vi "Test XYZ Table Stage Module All Axis.vi"() -> ()   [LabVIEW 2018]
uses:
  Hardware Mfg/Thorlabs Translation Stages/Controls/Translation Stage Cluster.ctl
  General/Controls/Translation Stage Types.ctl
  General/Controls/Translation Stage Parameters.ctl
  General/Controls/Set Get Controls.ctl
  Hardware Mfg/Thorlabs Translation Stages/Controls/Motion Translation Module Control.ctl
panel:
  in  "Table Stages":T1={"X Stage"={"Position"=0.0, "Is.Enabled?"=FALSE, "Is.Connected?"=FALSE, "Device SN"="45876425", "AccelerationMaximum"=0.0, "VelocityMaximum"=0.0, "Acceleration"=0.0, "Velocity"=0.0, "waitTimeout (ms)"=0, "Model"=enum."None", "Is.Homed?"=FALSE}, "Y Stage"={"Position"=0.0, "Is.Enabled?"=FALSE, "Is.Connected?"=FALSE, "Device SN"="45995820", "AccelerationMaximum"=0.0, "VelocityMaximum"=0.0, "Acceleration"=0.0, "Velocity"=0.0, "waitTimeout (ms)"=0, "Model"=enum."None", "Is.Homed?"=FALSE}, "Z Stage"={"Position"=0.0, "Is.Enabled?"=FALSE, "Is.Connected?"=FALSE, "Device SN"="49103464", "AccelerationMaximum"=0.0, "VelocityMaximum"=0.0, "Acceleration"=0.0, "Velocity"=0.0, "waitTimeout (ms)"=0, "Model"=enum."None", "Is.Homed?"=FALSE}}
  out "Cluster":T4
  in  "Z Pos":dbl caption="Position"
  in  "Y Pos":dbl caption="Position"
  in  "X Pos":dbl caption="Position"
  out "Error Out":errorcluster
  in  "Uninit":bool
  in  "Init":bool
  in  "Cancel Button":bool
  in  "Position":bool
  in  "Stop":bool
  in  "Home":bool
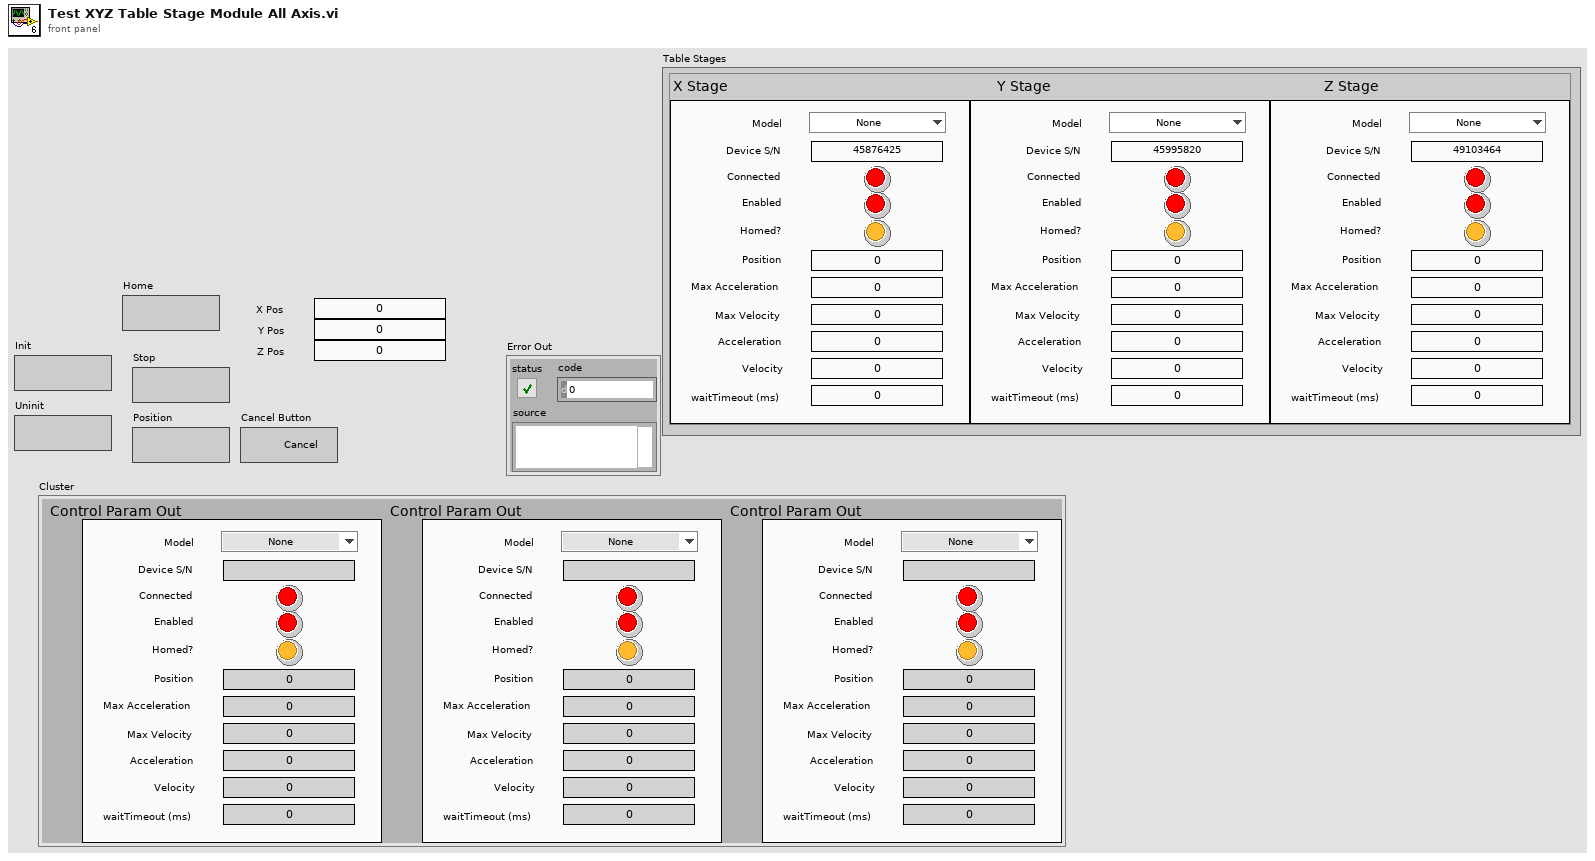
[diagram p1: front panel]
types:
  T1 = typedef "Translation Stage Parameters.ctl" = cluster{"X Stage":T2, "Y Stage":T2, "Z Stage":T2}
  T2 = typedef "Translation Stage Cluster.ctl" = cluster{"Position":dbl, "Is.Enabled?":bool, "Is.Connected?":bool, "Device SN":string, "AccelerationMaximum":dbl, "VelocityMaximum":dbl, "Acceleration":dbl, "Velocity":dbl, "waitTimeout (ms)":i32, "Model":T3, "Is.Homed?":bool}
  T3 = typedef "Translation Stage Types.ctl" = enum16{"None", "Thorlabs LTS", "Thorlabs MLJ"}
  T4 = cluster{"Control Param Out":T2, "Control Param Out":T2, "Control Param Out":T2}
  T5 = typedef "Motion Translation Module Control.ctl" = enum16{"Init", "Home", "Status", "Velocity/Accel", "Position", "Jog", "Stop", "Uninit", "Enable", "Disable"}
  T6 = typedef "Set Get Controls.ctl" = enum16{"Set", "Get"}
  T7 = typedef "System Parameters.ctl" = cluster{"Optical Parameters":T8, "Vibratome":T9, "Table Stages":T1, "Imaging Parameter":T10, "Galvo HW Parameters":cluster{"Analog Out Channel":tag, "Min Voltage":dbl, "Max Voltage":dbl, "Pixel Clock Source":tag, "Sample Rate":dbl, "Line Clock Out Ch":tag}, "Alazar parameters":T12, "Mosaic Paramter":cluster{"X Axis":cluster{"Start [mm]":dbl, "Steps [pts]":u16, "End [mm]":dbl}, "Y Axis":cluster{"Start [mm]":dbl, "Steps [pts]":u16, "End [mm]":dbl}, "Scan Pattern":enum16{"Uni-directional", "Bi-Directional", "Spiral Out", "Spiral In"}, "Overlap Options":cluster{"Overlap Type":enum16{"No Overlap", "X Only", "Y Only", "X and Y"}, "Percent Overlap":u8, "Justify":enum16{"Start", "Center", "End"}}}, "Vibratome Axis":cluster{"Start [mm]":dbl, "thick[mm]":dbl, "End [mm]":dbl}}
  T8 = typedef "Optical Parameters.ctl" = cluster{"Obj. Focal Length [mm]":dbl, "Scan Lens EFL[mm]":dbl, "Tube Lens EFL[mm]":dbl, "Galvo V Range (+/-)":dbl, "Galvo Max Half Angle [Deg]":dbl, "Max Galvo Range[%]":dbl}
  T9 = typedef "Vibratome Parameters.ctl" = cluster{"Z Bottom [mm]":dbl, "Pre Cut Dwell [s]":dbl, "Blade Frequency [RPM]":u16, "Slice Speed [mm/s]":dbl, "Post Cut Dwell [s]":dbl, "Ramp Time [s]":dbl, "Start X [mm]":dbl, "Start Y [mm]":dbl, "Slice Length [mm]":dbl, "Slice Axis":enum16{"X Axis", "Y Axis", "Z Axis"}, "Controller VISA Ref":refnum<visa-resource-name>}
  T10 = typedef "Imaging Parameters.ctl" = cluster{"Raster Scan Direction":T11, "Pixel Dwell Time [Clock Cycles]":u16, "Flyback Time [Clock Cycles]":u16, "XY Center [um]":cluster{"X":dbl, "Y":dbl}, "Pixel Step Size [um]":dbl, "XY Image Size":enum16{"32 x 32", "64 x 64", "128 x 128", "256 x 256", "512 x 512", "1024 x 1024", "2048 x 2048"}, "Custom":bool, "Custom Size":cluster{"X":u16, "Y":u16}, "Line Averages":u8}
  T11 = typedef "Scan Direction.ctl" = enum16{"Uni Directional", "Bi Directional", "None"}
  T12 = typedef "Alazar parameters.ctl" = cluster{"Trigger Settings":cluster{"General Trigger Settings":T13, "Trigger Engine 1":T14, "Trigger Engine 2":T14}, "Capture Clock":T15, "Device ID":T16, "Ch A Input Control":T17, "Ch B Input Control":T17, "Acq Settings":T18}
  T13 = typedef "General Trigger Settings.ctl" = cluster{"Trigger Operation":u32, "Coupling ID":u32, "Range ID":u32, "Delay":u32, "Timeout Ticks":u32, "Mode":u32, "Parameter":u32}
  T14 = typedef "Trigger Engine Controls.ctl" = cluster{"Trigger Engine":u32, "Source":u32, "Slope":u32, "Level":u32}
  T15 = typedef "Clock Controls.ctl" = cluster{"Sample Rate":u32, "Decimation":u32, "Source":u32, "Edge":u32}
  T16 = typedef "Alazar Device ID.ctl" = cluster{"System ID":u32, "Board ID":u32}
  T17 = typedef "Channel Input Controls.ctl" = cluster{"Channel":u8, "Coupling":u32, "Range":u32, "Impedance":u32}
  T18 = typedef "Alazar Acquisition Settings.ctl" = cluster{"Window Type":u32, "Record Length":u32, "Footer":u32, "Offset":u32, "Records Per Buffer":u32, "Samples per record":u32, "Records Count (Records/Acq)":u32, "Output Format":u32}
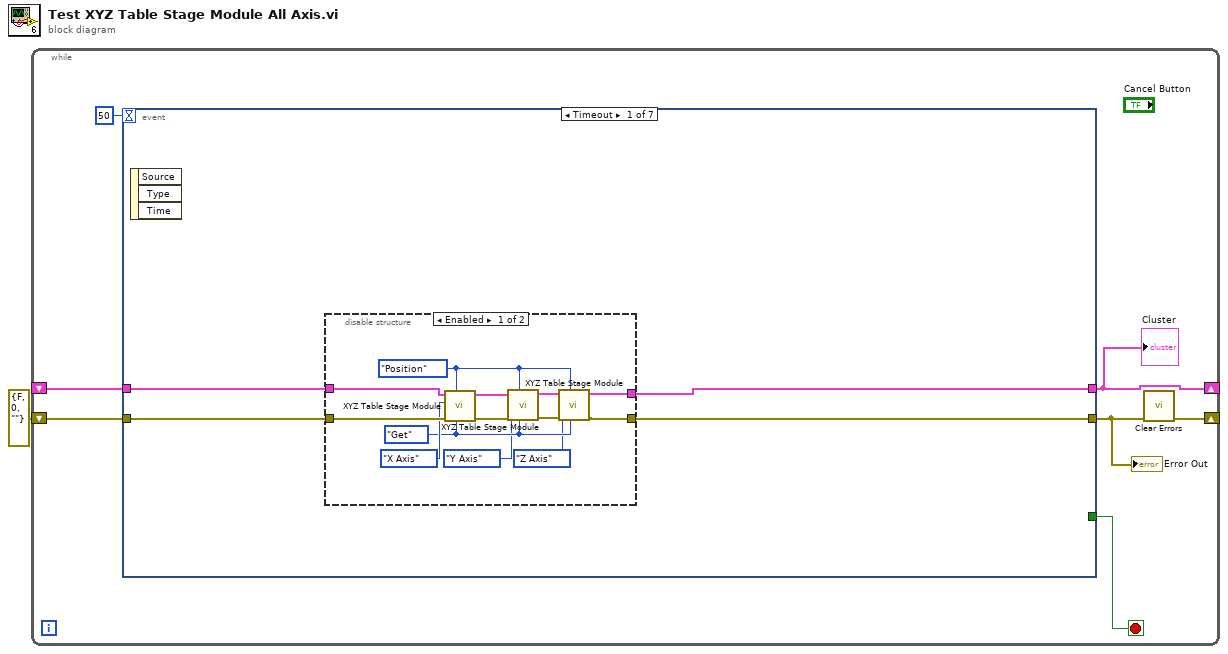
[diagram p0: block diagram]
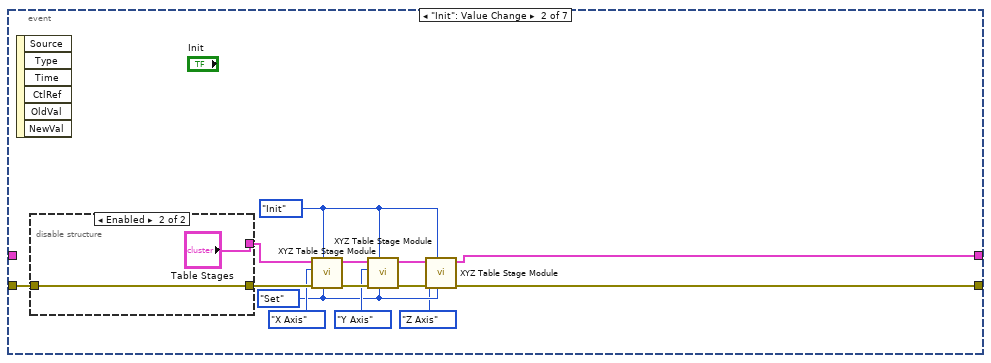
[diagram p3: hidden frame]
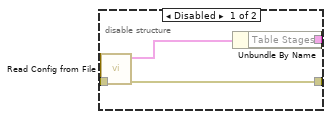
[diagram p4: hidden frame]
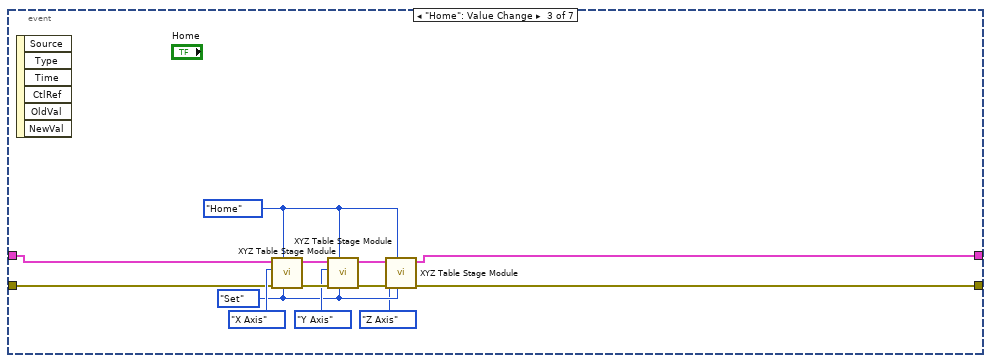
[diagram p5: hidden frame]
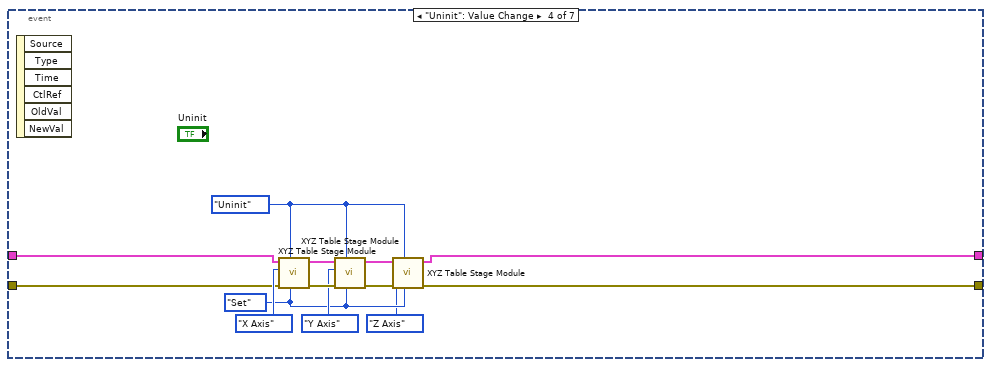
[diagram p6: hidden frame]
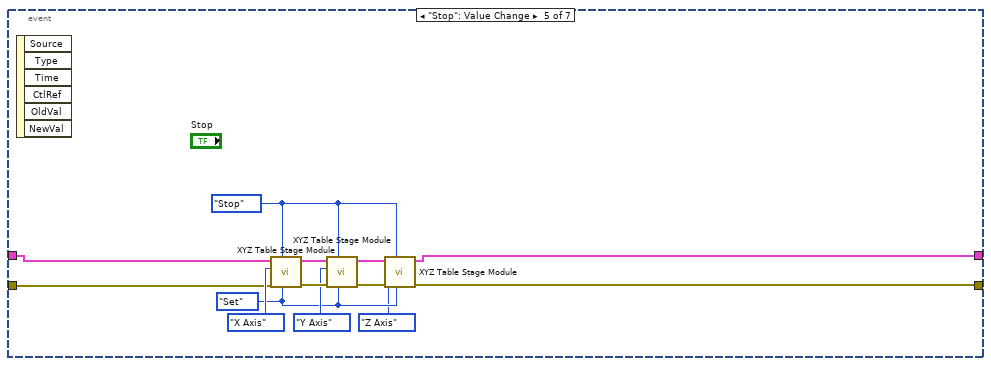
[diagram p7: hidden frame]
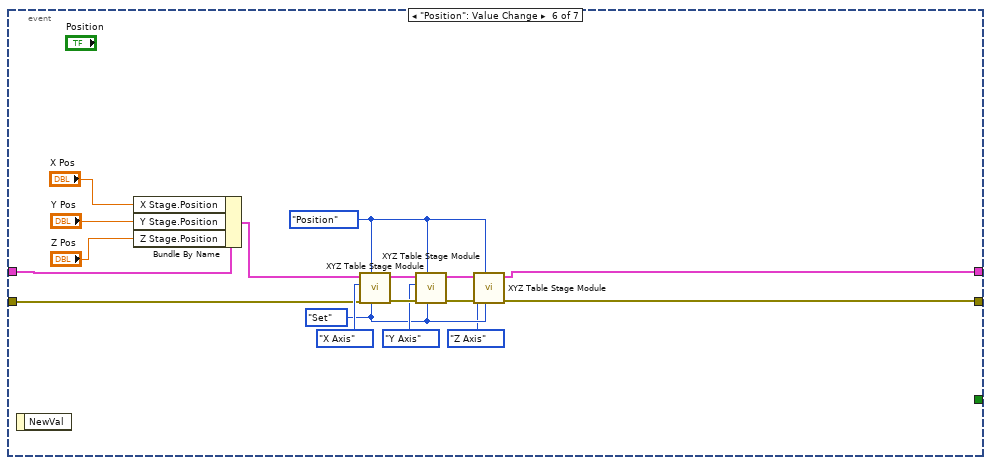
[diagram p8: hidden frame]
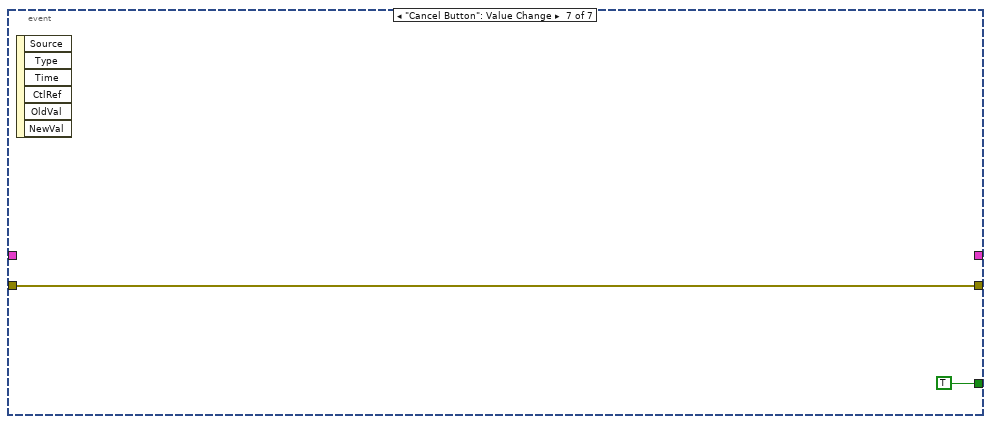
[diagram p9: hidden frame]
diagram:
  n1 = while {
    shift-right: [w3] -> _
    shift-left: errorcluster {"status"=FALSE, "code"=0, "source"=""} ("Error Out") -> [w5]
    shift-right: [w2] -> _
    shift-left: _ -> [w4]
    stop <- w7 stop-if-true
    n2 = event shown="[0] Timeout" {
      selector: _ -> [_ _ _ _ _ _ _]
      dyn-events: _ -> [_ _ _ _ _ _ _]
      timeout: 50 -> [_ _ _ _ _ _ _]
      tunnel: [_ _ _ _ _ _ TRUE] -> w7
      tunnel: [w9 w28 w48 w61 w74 w87 _] -> w2
      tunnel: w4 -> [w11 _ w51 w64 w77 w91 _]
      tunnel: [w10 w37 w52 w65 w78 w94 w104] -> w6
      tunnel: w5 -> [w12 w40 w53 w66 w79 w95 w104]
      event Timeout {
        n3 = event-data() -> ()  [unwired: 1 in, 3 out]
        n4 = disable-structure shown="Enabled" {
          disable-tunnel: w12 -> [w25 w26]
          disable-tunnel: w11 -> [w24 w27]
          disable-tunnel: [w14 w26] -> w10
          disable-tunnel: [w13 w27] -> w9
          frame Enabled {
            w18 = Motion_Translation_Module_Control."Position" ("Action")
            w17 = Set_Get_Controls."Get" ("Set/Get")
            n5 = call "XYZ Table Stage Module.vi"("Set/Get"=w17, "Action"=w18, "Error In"=w25, "Axis"=enum16{"X Axis", "Y Axis", "Z Axis"}."X Axis", "Table Stages"=w24) -> ("Error Out"=w20:errorcluster, "Table Stages [out]"=w19:T1)  [unwired: 5 in]
            n6 = call "XYZ Table Stage Module.vi"("Set/Get"=w17, "Action"=w18, "Error In"=w20, "Axis"=enum16{"X Axis", "Y Axis", "Z Axis"}."Y Axis", "Table Stages"=w19) -> ("Error Out"=w22:errorcluster, "Table Stages [out]"=w21:T1)  [unwired: 5 in]
            n7 = call "XYZ Table Stage Module.vi"("Set/Get"=w17, "Action"=w18, "Error In"=w22, "Axis"=enum16{"X Axis", "Y Axis", "Z Axis"}."Z Axis", "Table Stages"=w21) -> ("Error Out"=w14:errorcluster, "Table Stages [out]"=w13:T1)  [unwired: 5 in]
          }
          frame Disabled {
          }
        }
      }
      event "Init": Value Change {
        w34 = Set_Get_Controls."Set" ("Set/Get")
        w32 = Motion_Translation_Module_Control."Init" ("Action")
        n8 = event-data() -> ()  [unwired: 1 in, 6 out]
        n9 = disable-structure shown="Enabled" {
          disable-tunnel: w40 -> [w45 w47]
          disable-tunnel: [w44 w47] -> w39
          disable-tunnel: [w42 "Table Stages"] -> w31
          frame Disabled {
            n10 = call "Read Config from File.vi"("error in (no error)"=w45) -> ("error out"=w44:errorcluster, "System Parameters"=w43:T7)  [unwired: 9 in]
            n11 = Unbundle By Name(w43) -> ("Table Stages"=w42:T1)
          }
          frame Enabled {
          }
        }
        n12 = call "XYZ Table Stage Module.vi"("Set/Get"=w34, "Action"=w32, "Error In"=w39, "Axis"=enum16{"X Axis", "Y Axis", "Z Axis"}."X Axis", "Table Stages"=w31) -> ("Error Out"=w38:errorcluster, "Table Stages [out]"=w30:T1)  [unwired: 5 in]
        n13 = call "XYZ Table Stage Module.vi"("Set/Get"=w34, "Action"=w32, "Error In"=w38, "Axis"=enum16{"X Axis", "Y Axis", "Z Axis"}."Y Axis", "Table Stages"=w30) -> ("Error Out"=w41:errorcluster, "Table Stages [out]"=w29:T1)  [unwired: 5 in]
        n14 = call "XYZ Table Stage Module.vi"("Set/Get"=w34, "Action"=w32, "Error In"=w41, "Axis"=enum16{"X Axis", "Y Axis", "Z Axis"}."Z Axis", "Table Stages"=w29) -> ("Error Out"=w37:errorcluster, "Table Stages [out]"=w28:T1)  [unwired: 5 in]
      }
      event "Home": Value Change {
        w56 = Set_Get_Controls."Set" ("Set/Get")
        w54 = Motion_Translation_Module_Control."Home" ("Action")
        n15 = event-data() -> ()  [unwired: 1 in, 6 out]
        n16 = call "XYZ Table Stage Module.vi"("Set/Get"=w56, "Action"=w54, "Error In"=w53, "Axis"=enum16{"X Axis", "Y Axis", "Z Axis"}."X Axis", "Table Stages"=w51) -> ("Error Out"=w59:errorcluster, "Table Stages [out]"=w50:T1)  [unwired: 5 in]
        n17 = call "XYZ Table Stage Module.vi"("Set/Get"=w56, "Action"=w54, "Error In"=w59, "Axis"=enum16{"X Axis", "Y Axis", "Z Axis"}."Y Axis", "Table Stages"=w50) -> ("Error Out"=w60:errorcluster, "Table Stages [out]"=w49:T1)  [unwired: 5 in]
        n18 = call "XYZ Table Stage Module.vi"("Set/Get"=w56, "Action"=w54, "Error In"=w60, "Axis"=enum16{"X Axis", "Y Axis", "Z Axis"}."Z Axis", "Table Stages"=w49) -> ("Error Out"=w52:errorcluster, "Table Stages [out]"=w48:T1)  [unwired: 5 in]
      }
      event "Uninit": Value Change {
        w69 = Set_Get_Controls."Set" ("Set/Get")
        w67 = Motion_Translation_Module_Control."Uninit" ("Action")
        n19 = event-data() -> ()  [unwired: 1 in, 6 out]
        n20 = call "XYZ Table Stage Module.vi"("Set/Get"=w69, "Action"=w67, "Error In"=w66, "Axis"=enum16{"X Axis", "Y Axis", "Z Axis"}."X Axis", "Table Stages"=w64) -> ("Error Out"=w72:errorcluster, "Table Stages [out]"=w63:T1)  [unwired: 5 in]
        n21 = call "XYZ Table Stage Module.vi"("Set/Get"=w69, "Action"=w67, "Error In"=w72, "Axis"=enum16{"X Axis", "Y Axis", "Z Axis"}."Y Axis", "Table Stages"=w63) -> ("Error Out"=w73:errorcluster, "Table Stages [out]"=w62:T1)  [unwired: 5 in]
        n22 = call "XYZ Table Stage Module.vi"("Set/Get"=w69, "Action"=w67, "Error In"=w73, "Axis"=enum16{"X Axis", "Y Axis", "Z Axis"}."Z Axis", "Table Stages"=w62) -> ("Error Out"=w65:errorcluster, "Table Stages [out]"=w61:T1)  [unwired: 5 in]
      }
      event "Stop": Value Change {
        w82 = Set_Get_Controls."Set" ("Set/Get")
        w80 = Motion_Translation_Module_Control."Stop" ("Action")
        n23 = event-data() -> ()  [unwired: 1 in, 6 out]
        n24 = call "XYZ Table Stage Module.vi"("Set/Get"=w82, "Action"=w80, "Error In"=w79, "Axis"=enum16{"X Axis", "Y Axis", "Z Axis"}."X Axis", "Table Stages"=w77) -> ("Error Out"=w85:errorcluster, "Table Stages [out]"=w76:T1)  [unwired: 5 in]
        n25 = call "XYZ Table Stage Module.vi"("Set/Get"=w82, "Action"=w80, "Error In"=w85, "Axis"=enum16{"X Axis", "Y Axis", "Z Axis"}."Y Axis", "Table Stages"=w76) -> ("Error Out"=w86:errorcluster, "Table Stages [out]"=w75:T1)  [unwired: 5 in]
        n26 = call "XYZ Table Stage Module.vi"("Set/Get"=w82, "Action"=w80, "Error In"=w86, "Axis"=enum16{"X Axis", "Y Axis", "Z Axis"}."Z Axis", "Table Stages"=w75) -> ("Error Out"=w78:errorcluster, "Table Stages [out]"=w74:T1)  [unwired: 5 in]
      }
      event "Position": Value Change {
        w98 = Set_Get_Controls."Set" ("Set/Get")
        w96 = Motion_Translation_Module_Control."Position" ("Action")
        n27 = event-data() -> ()  [unwired: 1 in, 1 out]
        n28 = Bundle By Name(cluster=w91, "X Stage.Position"="X Pos", "Y Stage.Position"="Y Pos", "Z Stage.Position"="Z Pos") -> (w90:T1)
        n29 = call "XYZ Table Stage Module.vi"("Set/Get"=w98, "Action"=w96, "Error In"=w95, "Axis"=enum16{"X Axis", "Y Axis", "Z Axis"}."X Axis", "Table Stages"=w90) -> ("Error Out"=w101:errorcluster, "Table Stages [out]"=w89:T1)  [unwired: 5 in]
        n30 = call "XYZ Table Stage Module.vi"("Set/Get"=w98, "Action"=w96, "Error In"=w101, "Axis"=enum16{"X Axis", "Y Axis", "Z Axis"}."Y Axis", "Table Stages"=w89) -> ("Error Out"=w102:errorcluster, "Table Stages [out]"=w88:T1)  [unwired: 5 in]
        n31 = call "XYZ Table Stage Module.vi"("Set/Get"=w98, "Action"=w96, "Error In"=w102, "Axis"=enum16{"X Axis", "Y Axis", "Z Axis"}."Z Axis", "Table Stages"=w88) -> ("Error Out"=w94:errorcluster, "Table Stages [out]"=w87:T1)  [unwired: 5 in]
      }
      event "Cancel Button": Value Change {
        n32 = event-data() -> ()  [unwired: 1 in, 6 out]
      }
    }
    "Error Out" <- w6
    "Cluster" <- w2
    n33 = call <vilib>:"Clear Errors.vi"("error in (no error)"=w6) -> ("error out"=w3:errorcluster)  [unwired: 5 in, 1 out]
  }
